vi "Trash.vi"() -> ()   [LabVIEW 2015]
panel:
  in  "Trash full":dbl
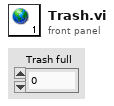
[diagram p1: front panel]
diagram:
